vi "nntcpautob.vi"() -> ()   [LabVIEW 2018, in "nn.lvlib"]
uses:
  nn.lvlib
panel:
  out "Signal":dynamicdata(graph) caption="Sine"
  out "Output":string
  out "Value":dbl
  out "Class":i32
  out "Training":bool
  in  "Port":u16=54321
  out "error out":errorcluster
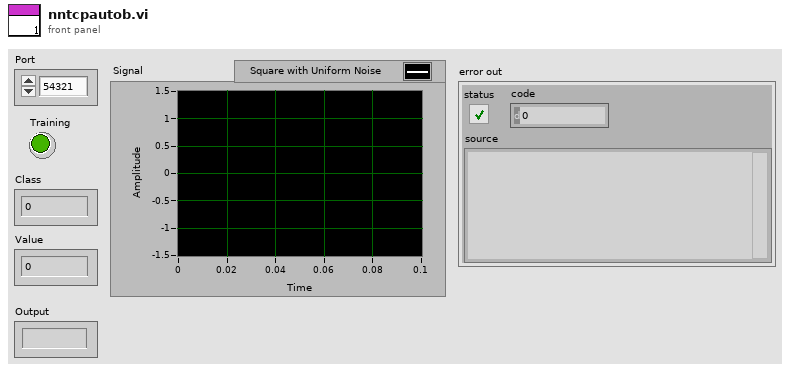
[diagram p1: front panel]
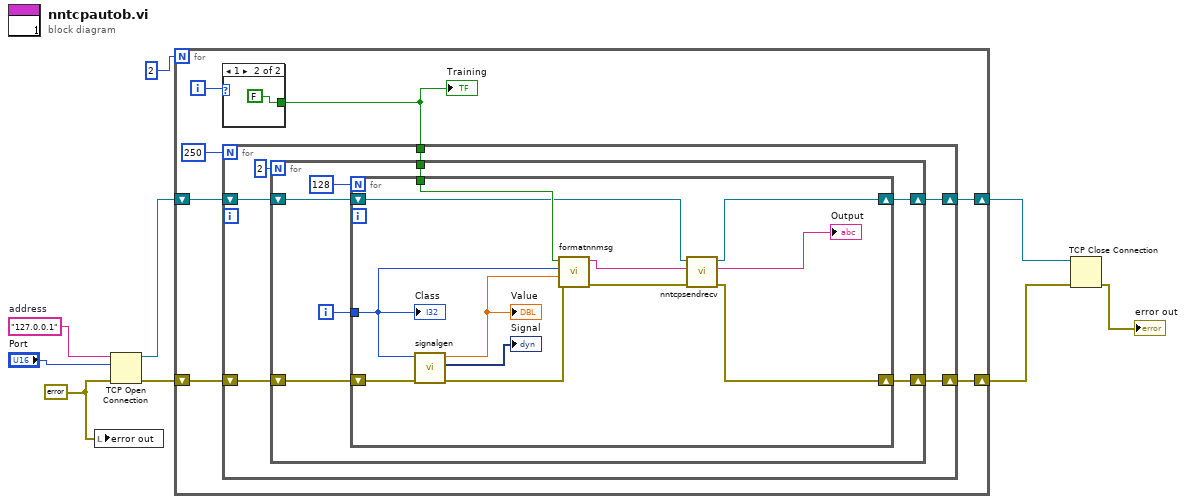
[diagram p0: block diagram]
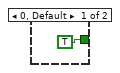
[diagram p2: hidden frame]
diagram:
  w8 = errorcluster {"status"=FALSE, "code"=0, "source"=""} ("error in (no error)")
  w6 = "127.0.0.1"  # address
  n1 = local write "error out"(w8) -> ()
  n2 = TCP Open Connection(address=w6, remote port or service name="Port", error in (no error)=w8) -> (connection ID=w2:refnum<k5>, error out=w4:errorcluster)  [unwired: 2 in]
  n3 = for {
    N: 2 -> [_]
    shift-right: [w13] -> w3
    shift-left: w4 -> [w14]
    shift-right: [w11] -> w1
    shift-left: w2 -> [w12]
    i -> [w16]
    n4 = case shown="1" w16 {
      tunnel: [TRUE FALSE] -> w10
      frame 0, Default {
      }
      frame 1 {
      }
    }
    "Training" <- w10
    n5 = for {
      N: 250 -> [_]
      tunnel: w10 -> [w21]
      shift-right: [w19] -> w13
      shift-left: w14 -> [w20]
      shift-right: [w17] -> w11
      shift-left: w12 -> [w18]
      n6 = for {
        N: 2 -> [_]
        tunnel: w21 -> [w26]
        shift-right: [w28] -> w19
        shift-left: w20 -> [w29]
        shift-right: [w23] -> w17
        shift-left: w18 -> [w27]
        i -> [w25]
        n7 = for {
          N: 128 -> [_]
          shift-right: [w32] -> w28
          shift-left: w29 -> [w35]
          shift-right: [w30] -> w23
          shift-left: w27 -> [w31]
          tunnel: w26 -> [w33]
          tunnel: w25 -> [w34]
          n8 = call "signalgen.vi"("error in (no error)"=w35, "Numeric in"=w34) -> ("error out"=w40:errorcluster, "Sawtooth"=→"Signal":dynamicdata, "Numeric out"=w38:dbl)  [unwired: 7 in]
          "Value" <- w38
          n9 = call "formatnnmsg.vi"("error in (no error)"=w40, "Numeric in"=w38, "Numeric"=w34, "Boolean"=w33) -> ("error out"=w37:errorcluster, "String"=w36:string)  [unwired: 6 in]
          n10 = call "nntcpsendrecv.vi"("error in (no error)"=w37, "String"=w36, "TCP Network Connection in"=w31) -> ("error out"=w32:errorcluster, "data out"=→"Output":string, "TCP Network Connection out"=w30:refnum<k5>)  [unwired: 6 in]
          "Class" <- w34
        }
      }
    }
  }
  n11 = TCP Close Connection(connection ID=w1, error in (no error)=w3) -> (error out=→"error out":errorcluster)  [unwired: 1 in, 1 out]
